vi "Use PID.vi"(8 "error in (no error)":errorcluster, 10 "X pixel translation":dbl format="%.2f", 11 "Retiga in":refnum<class "Retiga.lvclass">) -> (0 "error out":errorcluster, 2 "translation out":dbl, 3 "Retiga out":refnum<class "Retiga.lvclass">)   [LabVIEW 2012, in "Retiga.lvclass"]
uses:
  Retiga.lvclass
  Retiga.lvclass/Retiga.ctl
  <vilib>/addons/control/pid/pid.llb/PID (DBL).vi
  <vilib>/addons/control/pid/NI_PID_pid.lvlib
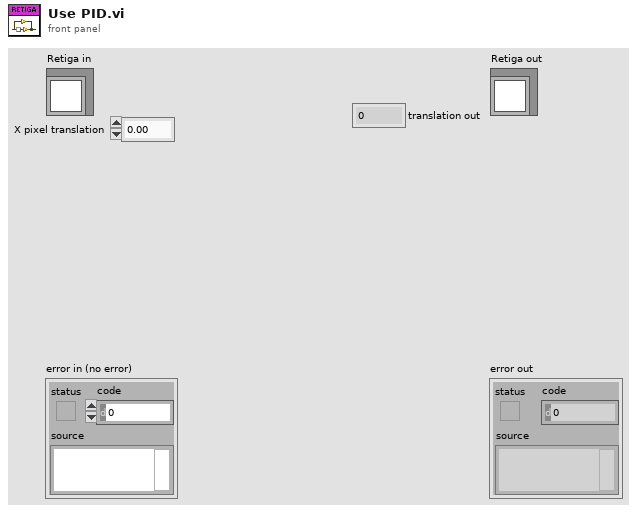
[diagram p1: front panel]
types:
  T1 = cluster{"proportional gain (Kc)":dbl, "integral time (Ti, min)":dbl, "derivative time (Td, min)":dbl}
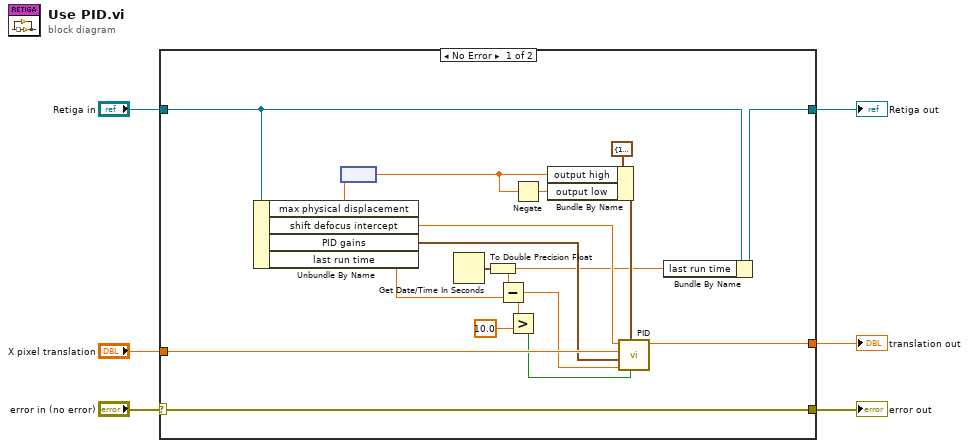
[diagram p0: block diagram]
diagram:
  n1 = case shown="No Error" "error in (no error)" {
    selector: "error in (no error)" -> [w24 w26]
    tunnel: [w24 w26] -> w5
    tunnel: [w7 w25] -> w3
    tunnel: "Retiga in" -> [w8 w25]
    tunnel: "X pixel translation" -> [w15 _]
    tunnel: [w10 _] -> w1
    frame No Error {
      n2 = Unbundle By Name(w8) -> ("max physical displacement"=w17:dbl[unit], "shift defocus intercept"=w16:dbl, "PID gains"=w14:T1, "last run time"=w13:dbl)
      n3 = node(w17) -> (w18:dbl)
      n4 = Get Date/Time In Seconds() -> (seconds since 1Jan1904=w23:timestamp)
      n5 = To Double Precision Float(number=w23) -> (double precision float=w9:dbl)
      n6 = Subtract(x=w9, y=w13) -> (x-y=w12:dbl)
      n7 = Greater?(x=w12, y=10.0) -> (0:w11:bool)
      n8 = Negate(x=w18) -> (-x=w19:dbl)
      n9 = Bundle By Name(cluster=cluster{"output high":dbl, "output low":dbl} {"output high"=100.0, "output low"=-100.0} ("output range"), "output high"=w18, "output low"=w19) -> (w20:cluster{"output high":dbl, "output low":dbl})
      n10 = call-poly <vilib>:"PID.vi"("reinitialize? (F)"=w11, "output range"=w20, "dt (s)"=w12, "PID gains"=w14, "process variable"=w15, "setpoint"=w16) -> ("output"=w10:dbl)  [unwired: 4 in, 1 out]
      n11 = Bundle By Name(cluster=w8, "last run time"=w9) -> (w7:refnum<class "Retiga.lvclass">)
    }
    frame Error {
    }
  }
  "error out" <- w5
  "Retiga out" <- w3
  "translation out" <- w1
